vi "main.vi"() -> ()   [LabVIEW 2020]
uses:
  <vilib>/vision/Image Controls.llb/IMAQ Image.ctl
panel:
  in  "write buffer":string
  in  "TestBaud":u32=115200
  in  "TestPort":refnum<visa-resource-name>="COM6"
  out "TestReceivingFromSTM":string
  in  "Baud":u32=115200
  in  "Port":refnum<visa-resource-name>="COM6"
  out "ReceivingFromSTM":string
  in  "Recognise":bool
  in  "Process":bool
  in  "Stop acquisition":bool
  in  "Acquire":bool
  out "Image":T1(plugin-control)
  in  "Stop program":bool
  # "Serwo_Test"
  # "First Press \"Acquire\""
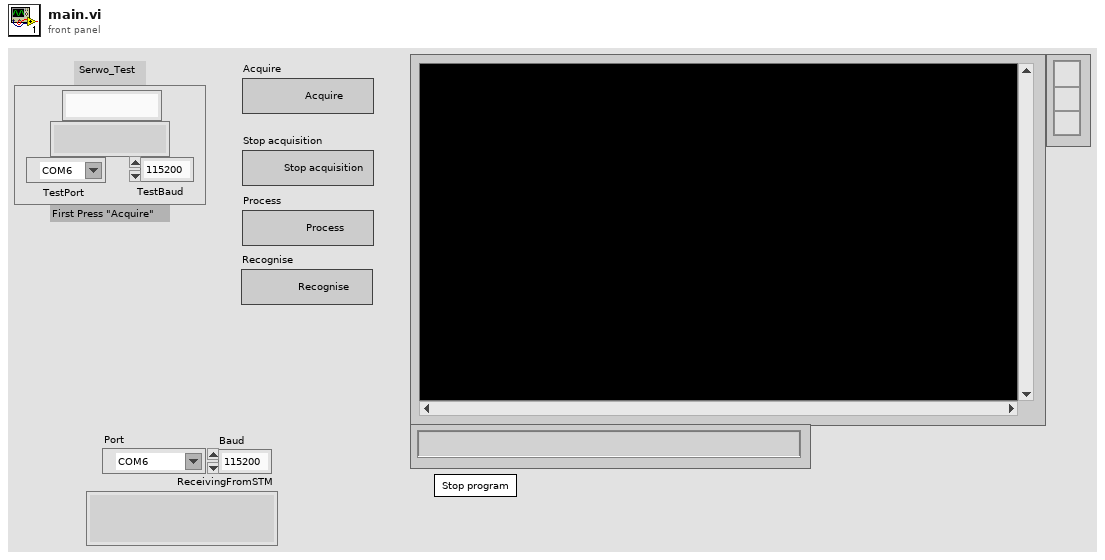
[diagram p1: front panel]
types:
  T1 = typedef "IMAQ Image.ctl" = refnum<image>
  T2 = enum32{"Invalid", "Standard", "Closed", "Hidden", "Minimized", "Maximized"}
  T3 = enum32{"invalid app kind", "Development System", "Run Time System", "Student Edition", "Embedded LabVIEW", "Evaluation", "Custom"}
  T4 = cluster{"Core":cluster{"Current VI Reference":refnum<vi>, "Close Panel on Exit?":bool}, "Aborted":bool, "New Image":T1, "Processing":bool, "Recognising":bool}
  T5 = cluster{"Current VI Reference":refnum<vi>, "Close Panel on Exit?":bool}
  T6 = typedef "Image Type" = u32
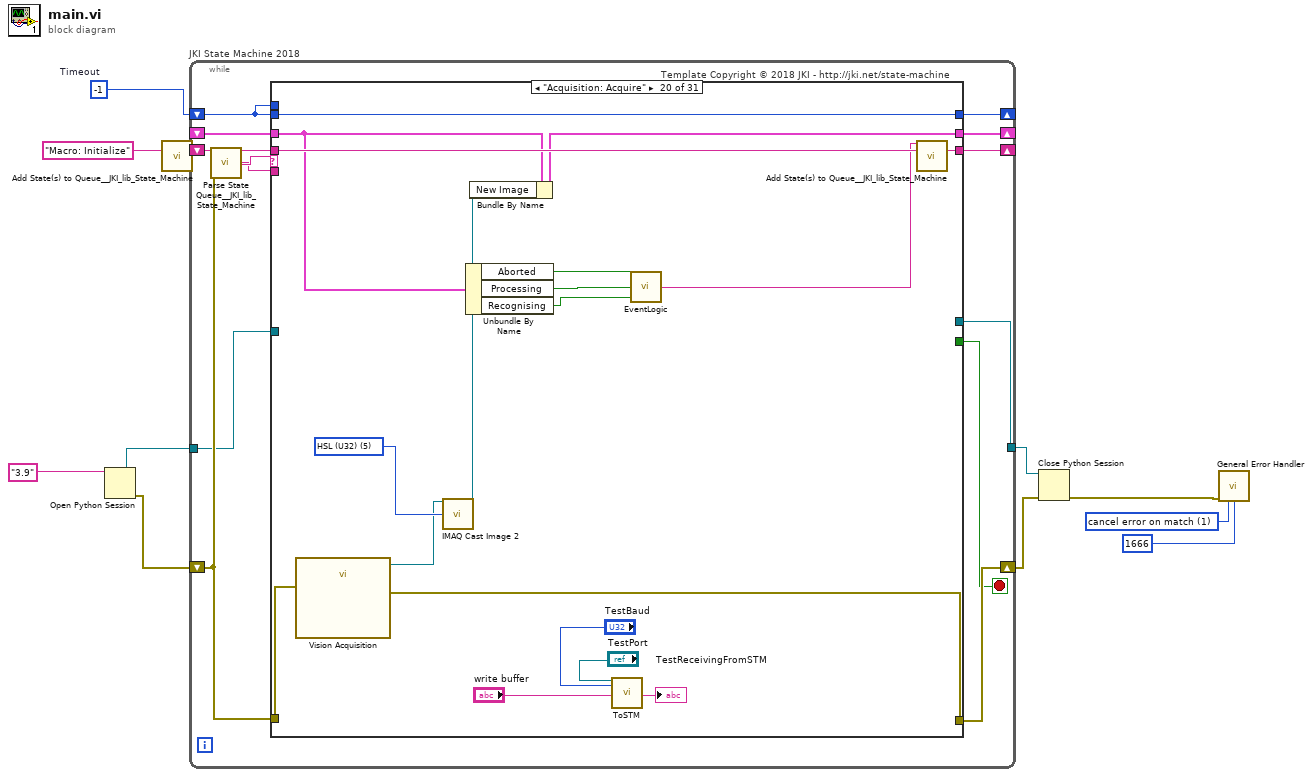
[diagram p0: block diagram]
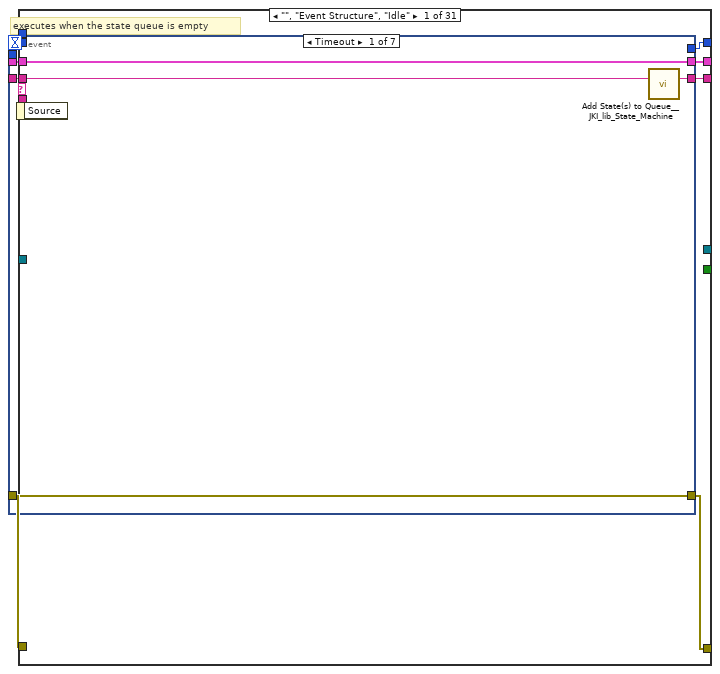
[diagram p2: hidden frame]
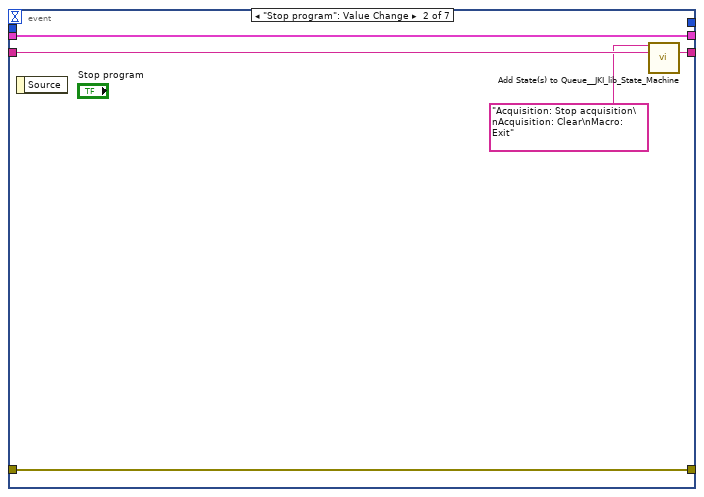
[diagram p3: hidden frame]
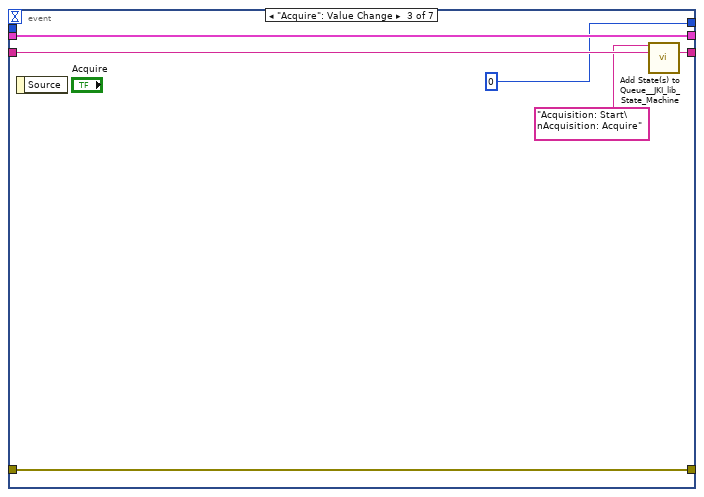
[diagram p4: hidden frame]
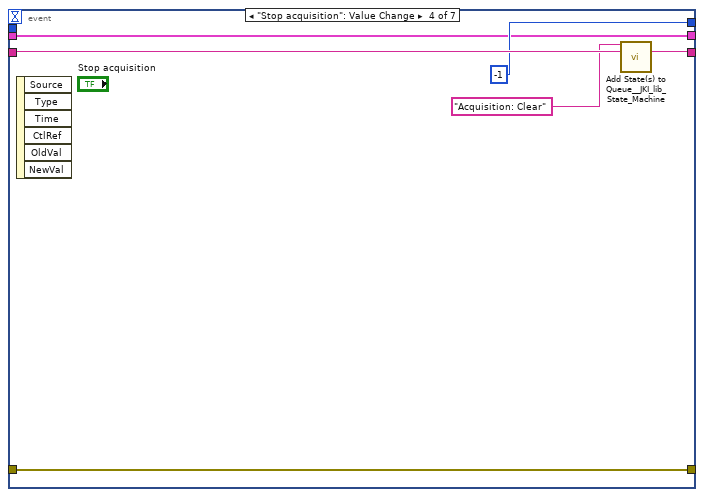
[diagram p5: hidden frame]
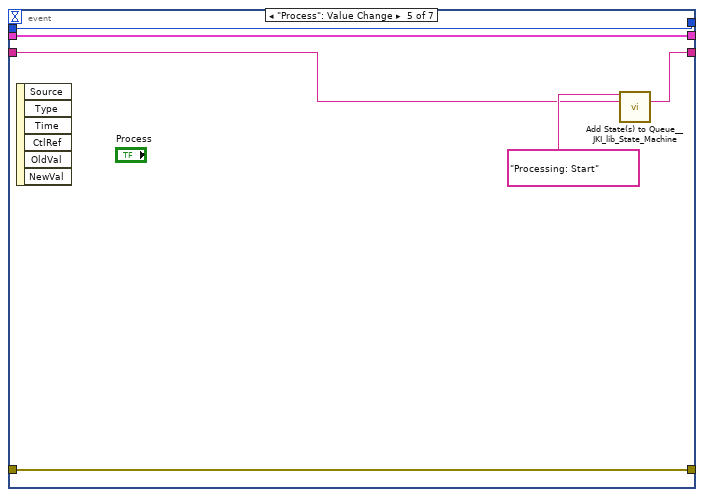
[diagram p6: hidden frame]
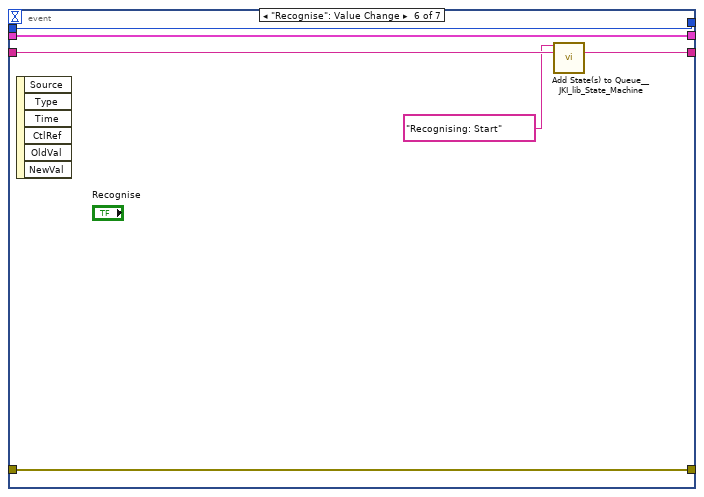
[diagram p7: hidden frame]
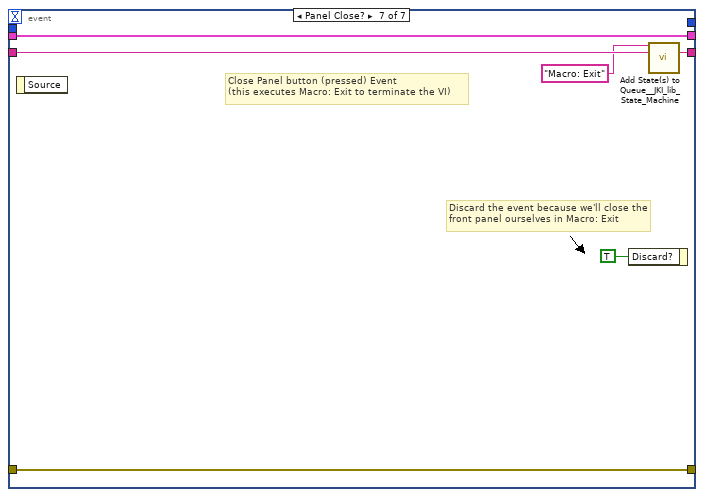
[diagram p8: hidden frame]
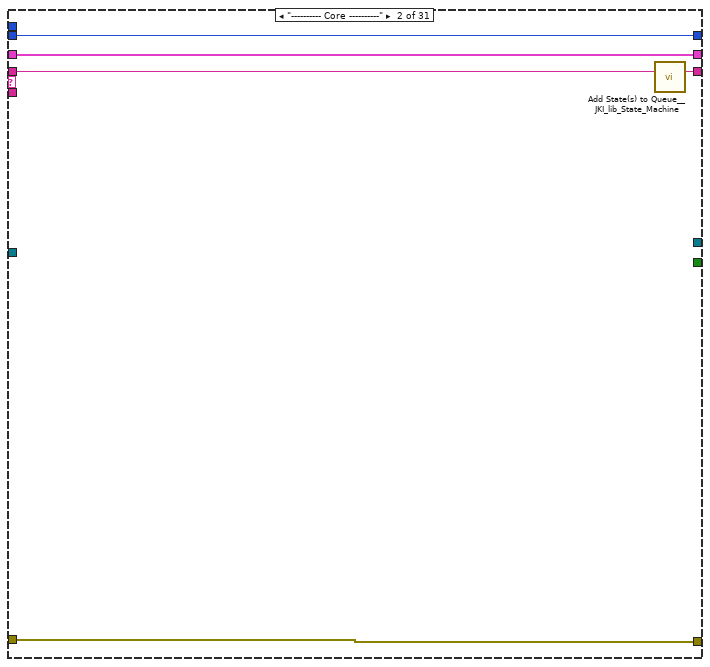
[diagram p9: hidden frame]
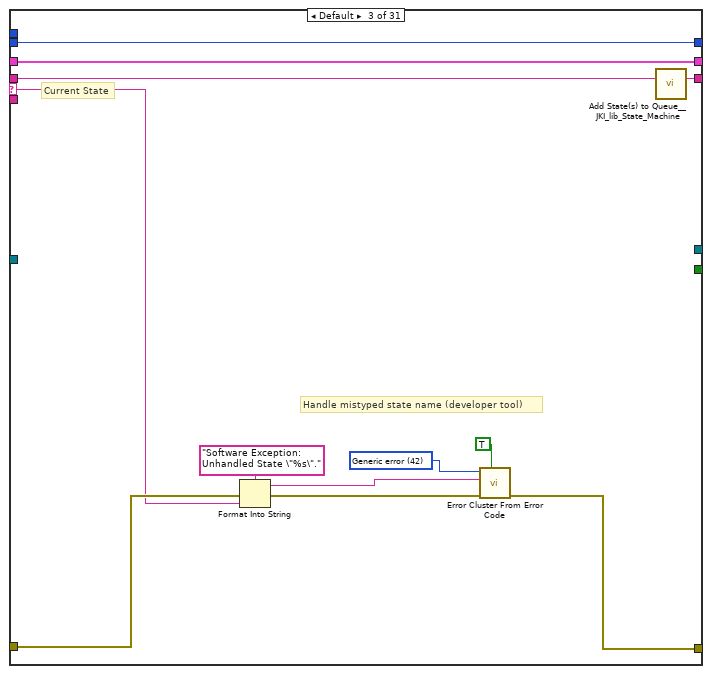
[diagram p10: hidden frame]
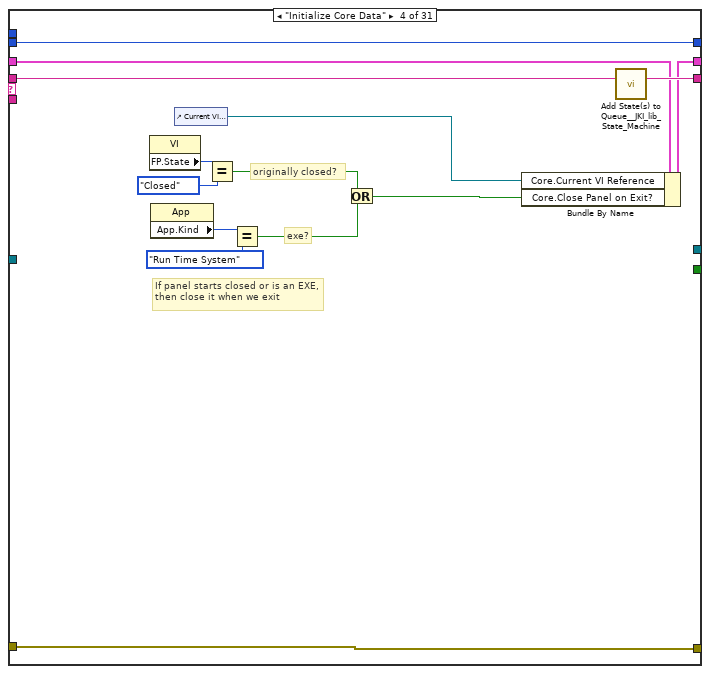
[diagram p11: hidden frame]
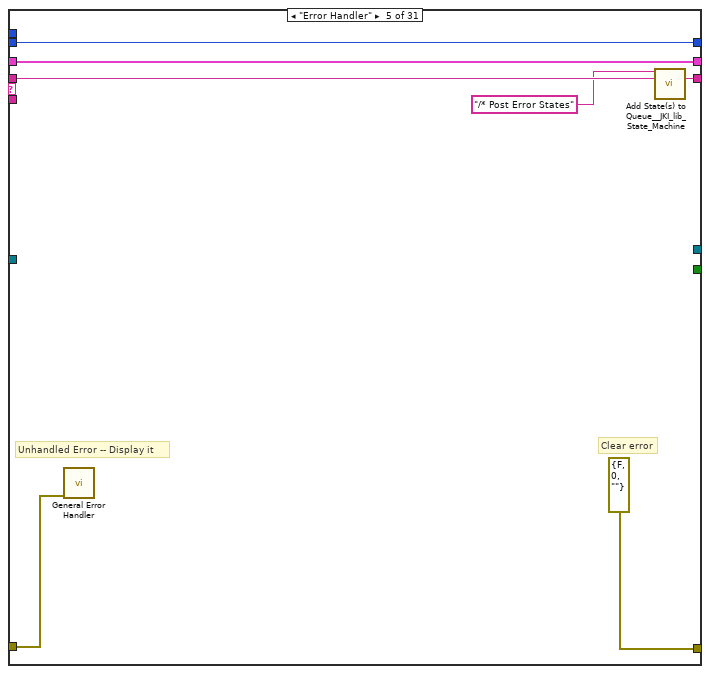
[diagram p12: hidden frame]
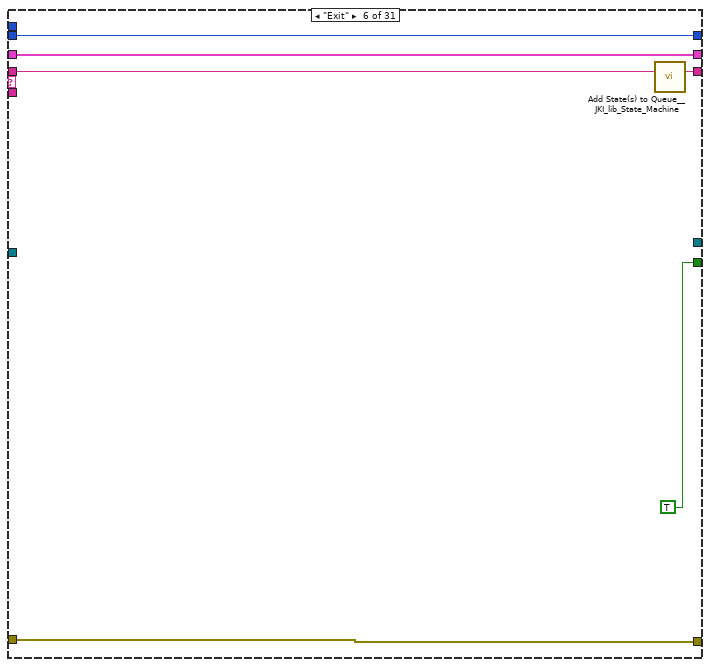
[diagram p13: hidden frame]
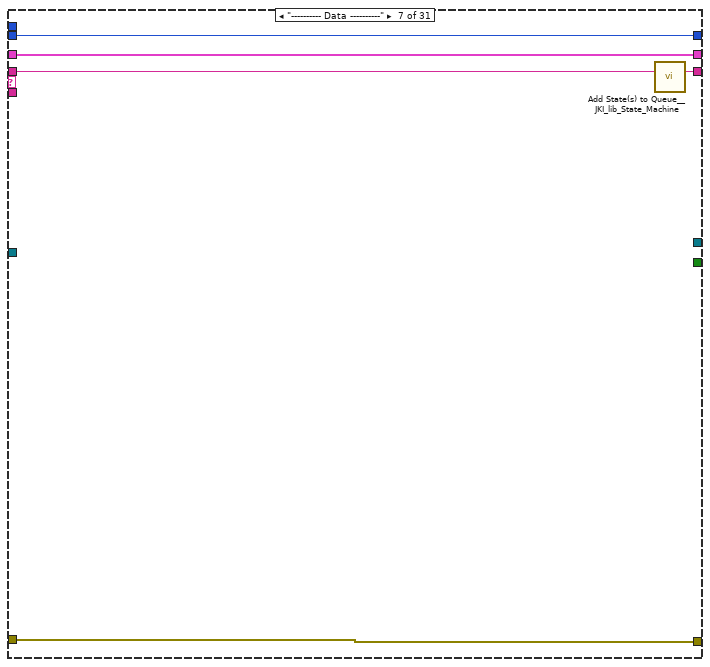
[diagram p14: hidden frame]
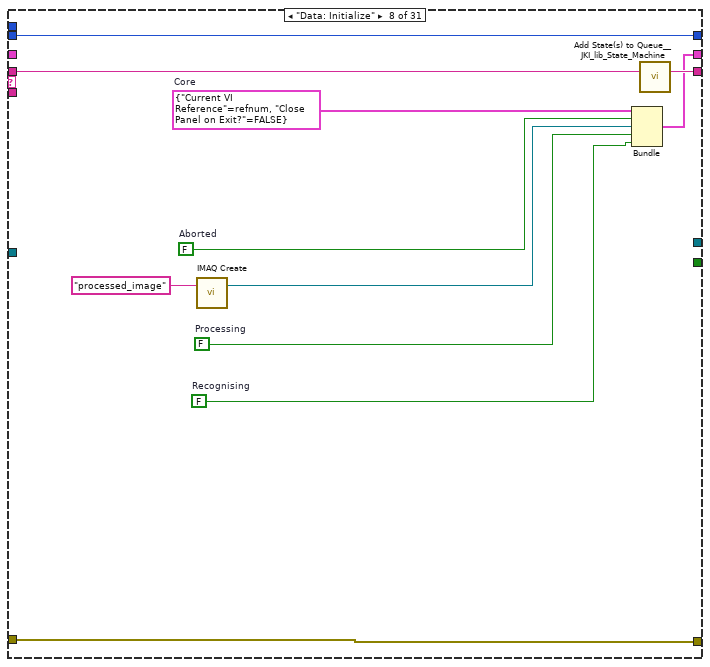
[diagram p15: hidden frame]
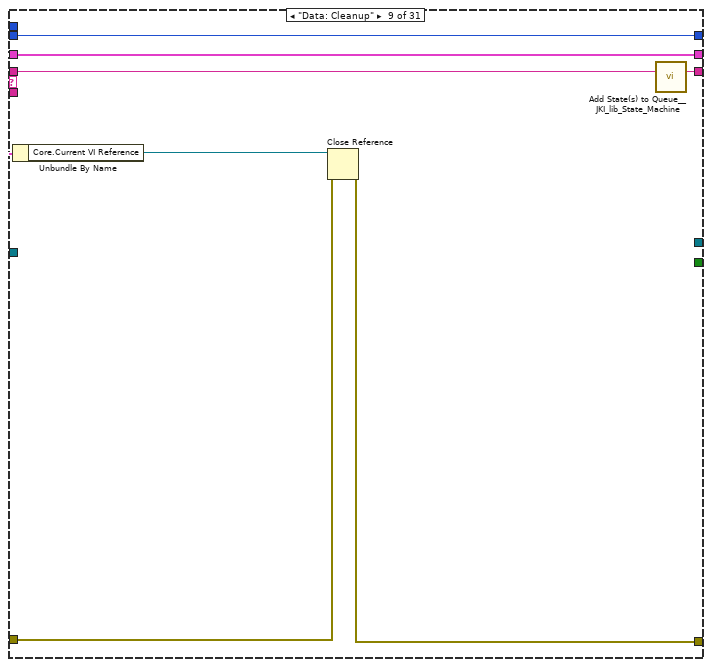
[diagram p16: hidden frame]
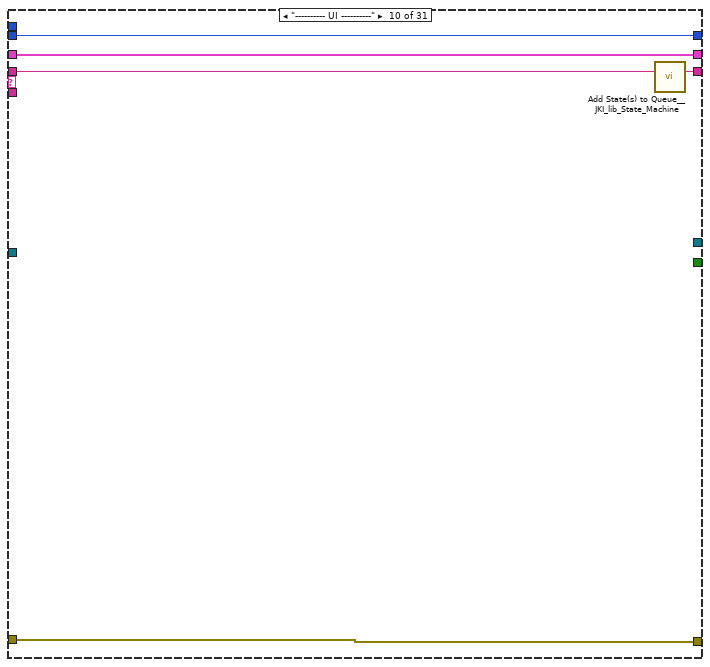
[diagram p17: hidden frame]
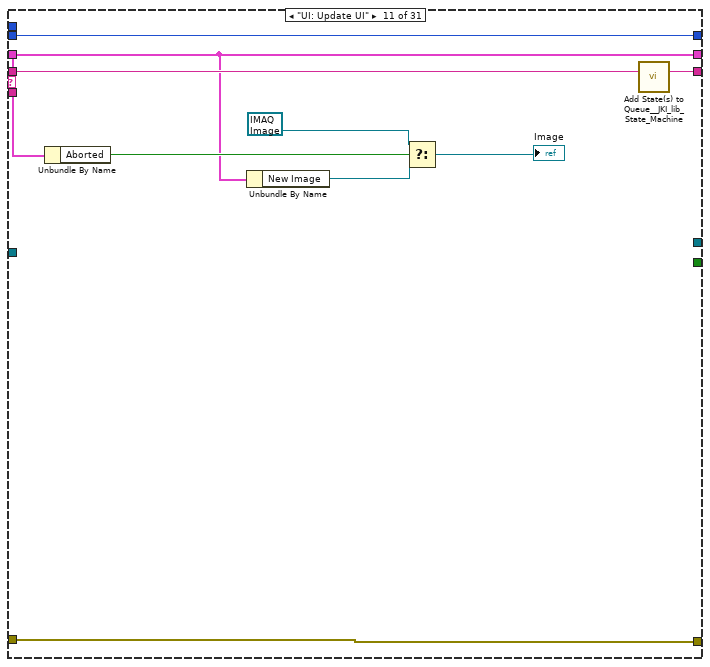
[diagram p18: hidden frame]
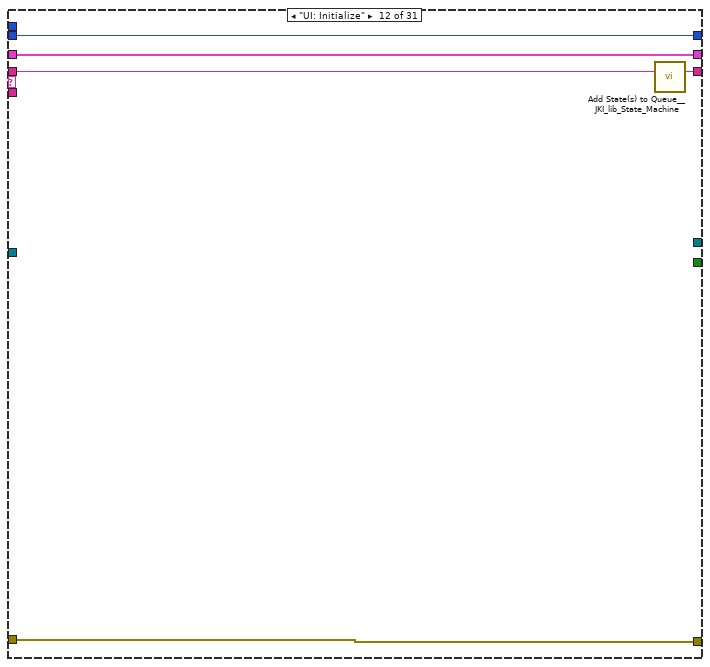
[diagram p19: hidden frame]
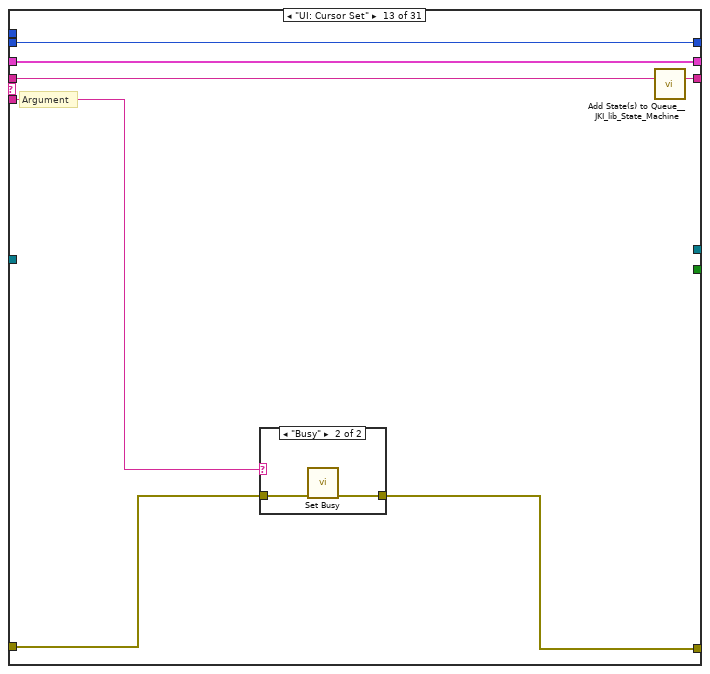
[diagram p20: hidden frame]
diagram:
  w3 = 1 items=["no exception", "cancel error on match", "set error on match"] ("[exception action] (none:0)")
  w9 = -1  # Timeout
  n1 = Open Python Session(python version="3.9" ("Python version")) -> (session out=w8:refnum<k35>, error out=w6:errorcluster)  [unwired: 2 in]
  n2 = call <vilib>:"Add State(s) to Queue__JKI_lib_State_Machine.vi"("State(s) in (\"\")"="Macro: Initialize") -> ("States Out"=w11:string)  [unwired: 14 in]
  n3 = while "JKI State Machine 2018" {
    shift-right: [w18] -> _
    shift-left: _ -> [w17]
    shift-right: [w21] -> w4
    shift-left: w6 -> [w16]
    shift-right: [w20] -> _
    shift-left: w11 -> [w22]
    shift-right: [w15] -> _
    shift-left: w9 -> [w14]
    tunnel: w8 -> [w13]
    tunnel: [w12] -> w5
    stop <- w19 stop-if-true
    # "Template Copyright © 2018 JKI - http://jki.net/state-machine"
    n4 = call <vilib>:"Parse State Queue__JKI_lib_State_Machine.vi"("State Queue"=w22, "Error In (no error)"=w16) -> ("Remaining States"=w24:string, "Current State"=w25:string, "Arguments"=w23:string)  [unwired: 11 in]
    n5 = case shown="\"Acquisition: Acquire\"" w25 {
      selector: w25 -> [_ _ w79 _ _ _ _ _ _ _ _ _ _ _ _ _ _ _ _ _ _ _ _ _ _ _ _ _ _ _ _]
      tunnel: w24 -> [w33 w77 w83 w103 w110 w116 w121 w132 w139 w144 w152 w158 w165 w177 w247 w253 w264 w269 w276 w294 w301 w310 w315 w320 w327 w347 w352 w357 w364 w386 w391]
      tunnel: w23 -> [_ _ _ _ _ _ _ _ _ _ _ _ w160 w171 _ _ _ _ _ _ _ _ _ _ _ _ _ _ _ _ _]
      tunnel: w17 -> [w31 w74 w81 w96 w107 w114 w118 _ w134 w141 w148 w156 w163 w173 w244 w250 w261 w266 w271 w292 w297 w306 w312 w317 w323 w343 w349 w354 w360 w371 w388]
      tunnel: [w30 w75 w85 w100 errorcluster {"status"=FALSE, "code"=0, "source"=""} ("error out") w113 w119 w129 w135 w142 w146 w155 w161 w174 w245 w251 w262 w267 w274 w286 w299 w308 w313 w318 w325 w336 w350 w355 w362 w370 w389] -> w21
      tunnel: w16 -> [w29 w75 w84 w100 w106 w113 w119 w129 w136 w142 w146 w155 w162 w175 w245 w251 w262 w267 w274 w282 w299 w308 w313 w318 w325 w335 w350 w355 w362 w373 w389]
      tunnel: [w32 w76 w82 w102 w109 w115 w120 w131 w138 w143 w153 w157 w164 w176 w246 w252 w263 w268 w275 w293 w300 w309 w314 w319 w326 w346 w351 w356 w363 w385 w390] -> w20
      tunnel: [_ _ _ _ _ TRUE _ _ _ _ _ _ _ _ _ _ _ _ _ _ _ _ _ _ _ _ _ _ _ _ _] -> w19
      tunnel: [w28 w74 w81 w101 w107 w114 w118 w130 w134 w141 w148 w156 w163 w173 w244 w250 w261 w266 w272 w291 w296 w306 w312 w317 w322 w342 w349 w354 w359 w371 w388] -> w18
      tunnel: w14 -> [w26 w73 _ w90 w104 w111 w117 w125 w133 w140 w145 w154 w159 w170 w243 w248 w254 w265 w270 w287 w298 w307 w311 w316 w324 w345 w348 w353 w361 w384 w387]
      tunnel: [w27 w73 w78 w90 w104 w111 w117 w125 w133 w140 w145 w154 w159 w170 w243 w248 w254 w265 w270 w287 w298 w307 w311 w316 w324 w345 w348 w353 w361 w384 w387] -> w15
      tunnel: w14 -> [_ _ w78 _ _ _ _ _ _ _ _ _ _ _ _ _ _ _ _ _ _ _ _ _ _ _ _ _ _ _ _]
      tunnel: w13 -> [_ _ _ _ _ _ _ _ _ _ _ _ _ _ _ _ _ _ _ _ _ _ _ _ _ w329 _ _ _ w372 _]
      tunnel: [_ _ _ _ _ _ _ _ _ _ _ _ _ _ _ _ _ _ _ _ _ _ _ _ _ w328 _ _ _ w368 _] -> w12
      frame "", "Event Structure", "Idle" {
        # "executes when the state queue is empty"
        n6 = event shown="[0] Timeout" {
          selector: _ -> [_ _ _ _ _ _ _]
          dyn-events: _ -> [_ _ _ _ _ _ _]
          timeout: w26 -> [_ _ _ _ _ _ _]
          tunnel: w33 -> [w37 w42 w48 w53 w55 w65 w72]
          tunnel: [w36 w41 w47 w54 w59 w63 w71] -> w32
          tunnel: w31 -> [w34 w39 w45 w50 w60 w66 w69]
          tunnel: [w35 w40 w46 w49 w56 w62 w70] -> w30
          tunnel: w29 -> [w35 w40 w46 w49 w56 w62 w70]
          tunnel: [w34 w39 w45 w50 w60 w66 w69] -> w28
          tunnel: [_ _ 0 ("Timeout") -1 ("Timeout") w57 w61 _] -> w27
          tunnel: w26 -> [_ _ _ _ w57 w61 _]
          event Timeout {
            n7 = event-data() -> ()  [unwired: 1 in, 1 out]
            n8 = call <vilib>:"Add State(s) to Queue__JKI_lib_State_Machine.vi"("State(s) in (\"\")"=w37) -> ("States Out"=w36:string)  [unwired: 14 in]
          }
          event "Stop program": Value Change {
            n9 = event-data() -> ()  [unwired: 1 in, 1 out]
            n10 = call <vilib>:"Add State(s) to Queue__JKI_lib_State_Machine.vi"("State(s) in Front (\"\")"="Acquisition: Stop acquisition\nAcquisition: Clear\nMacro: Exit", "State(s) in (\"\")"=w42) -> ("States Out"=w41:string)  [unwired: 13 in]
          }
          event "Acquire": Value Change {
            n11 = event-data() -> ()  [unwired: 1 in, 1 out]
            n12 = call <vilib>:"Add State(s) to Queue__JKI_lib_State_Machine.vi"("State(s) in Front (\"\")"="Acquisition: Start\nAcquisition: Acquire", "State(s) in (\"\")"=w48) -> ("States Out"=w47:string)  [unwired: 13 in]
          }
          event "Stop acquisition": Value Change {
            n13 = event-data() -> ()  [unwired: 1 in, 6 out]
            n14 = call <vilib>:"Add State(s) to Queue__JKI_lib_State_Machine.vi"("State(s) in Front (\"\")"="Acquisition: Clear" ("State(s) in Front (\"\")"), "State(s) in (\"\")"=w53) -> ("States Out"=w54:string)  [unwired: 13 in]
          }
          event "Process": Value Change {
            n15 = event-data() -> ()  [unwired: 1 in, 6 out]
            n16 = call <vilib>:"Add State(s) to Queue__JKI_lib_State_Machine.vi"("State(s) in Front (\"\")"="Processing: Start" ("State(s) in Front (\"\")"), "State(s) in (\"\")"=w55) -> ("States Out"=w59:string)  [unwired: 13 in]
          }
          event "Recognise": Value Change {
            n17 = event-data() -> ()  [unwired: 1 in, 6 out]
            n18 = call <vilib>:"Add State(s) to Queue__JKI_lib_State_Machine.vi"("State(s) in Front (\"\")"="Recognising: Start" ("State(s) in Front (\"\")"), "State(s) in (\"\")"=w65) -> ("States Out"=w63:string)  [unwired: 13 in]
          }
          event Panel Close? {
            # "Discard the event because we'll close the front panel ourselves in Macro: Exit"
            # "Close Panel button (pressed) Event\n(this executes Macro: Exit to terminate the VI)"
            n19 = event-data() -> ()  [unwired: 1 in, 1 out]
            n20 = event-data("Discard?"=TRUE) -> ()  [unwired: 1 in, 1 out]
            n21 = call <vilib>:"Add State(s) to Queue__JKI_lib_State_Machine.vi"("State(s) in Front (\"\")"="Macro: Exit", "State(s) in (\"\")"=w72) -> ("States Out"=w71:string)  [unwired: 13 in]
          }
        }
      }
      frame "---------- Core ----------" {
        n22 = call <vilib>:"Add State(s) to Queue__JKI_lib_State_Machine.vi"("State(s) in (\"\")"=w77) -> ("States Out"=w76:string)  [unwired: 14 in]
      }
      frame Default {
        w88 = 42 items=["No error", "Argument error", "Memory is full", "Out of zone", "End of file", "File already open", "Generic file I/O error", "File not found", "File permission error", "Disk is full", "Duplicate path", "Too many files open", "System feature not enabled", "Resource file not found", "Cannot add resource", "Resource not found", "Image not found", "Image memory error", "Pen does not exist", "Config type invalid", "Config token not found", "Config parse error", "Config memory error", "Bad external code format", "Bad external code offset", "External code not present", "Null window", "Destroy window error", "Null menu", "Print aborted", "Bad print record", "Print driver error", "Windows error during printing", "Memory error during printing", "Print dialog error", "Generic print error", "Invalid device refnum", "Device not found", "Device parameter error", "Device unit error", "Cannot open device", "Device call aborted", "Generic error", "Cancelled by user", "Object ID too low", "Object ID too high", "Object not in heap", "Unknown heap", "Unknown object (invalid DefProc)", "Unknown object (DefProc not in table)", "Message out of range", "Invalid (null) method", "Unknown message", "Manager call not supported", "Bad address", "Network operation in progress", "Network operation timed out", "Connection is busy", "Network attribute not supported", "Network error", "Address in use", "System out of memory", "Connection aborted", "Connection refused", "Not connected", "Already connected", "Connection closed", "Initialization error (interapplication manager)", "Bad occurrence", "Wait on unbound occurrence handler", "Occurrence queue overflow", "Datalog type conflict", "Unused", "Unrecognized type (interapplication manager)", "Memory corrupt", "Failed to make temporary DLL", "Old CIN version", "Drag socket not found", "Failed to load drop-object", "Failed to register OLE object", "Failed to release OLE object", "Format specifier type mismatch", "Unknown format specifier", "Too few format specifiers", "Too many format specifiers", "Scan failed", "Newer CIN version", "Error converting to variant", "Runtime menu error", "Password tampered", "Variant attribute not found", "Incompatible variant data type", "Event data is not available", "Event Store is not present", "Occurrence is not found", "Event Queue is not created", "Event info is not available", "Refnum passed is NULL", "Error retrieving Class GUID", "Error retrieving CoClass GUID", "Error retrieving TypeLib GUID.", "Bad built application magic bytes.", "Specific driver is different from the specific driver associated with the Logical Name.", "There is no session opened to the class driver.", "Max Error", "MAX - Error with config objects", "MAX - Error loading configuration", "MAX - Group not supported"]
        # "Current State"
        # "Handle mistyped state name (developer tool)"
        n23 = Format Into String(format string="Software Exception: Unhandled State \"%s\"." ("message"), error in=w84, w79) -> (resulting string=w87:string, error out=w86:errorcluster)  [unwired: 1 in]
        n24 = call <vilib>:"Error Cluster From Error Code.vi"("show call chain? (False)"=TRUE, "error in (no error)"=w86, "error message (\"\")"=w87, "error code (0)"=w88) -> ("error out"=w85:errorcluster)  [unwired: 5 in]
        n25 = call <vilib>:"Add State(s) to Queue__JKI_lib_State_Machine.vi"("State(s) in (\"\")"=w83) -> ("States Out"=w82:string)  [unwired: 14 in]
      }
      frame "Initialize Core Data" {
        # "originally closed?"
        # "exe?"
        # "If panel starts closed or is an EXE, then close it when we exit"
        n26 = property class="VI"() -> ("FP.State"=w93:T2)  [unwired: 2 in, 2 out]
        n27 = property class="App"() -> ("App.Kind"=w99:T3)  [unwired: 2 in, 2 out]
        n28 = control-ref of="Current VI Reference"() -> (w94:refnum<vi>)
        n29 = Equal?(x=w93, y=T2."Closed" ("Front Panel Window:State")) -> (x = y?=w91:bool)
        n30 = Equal?(x=w99, y=T3."Run Time System" ("Application:Kind")) -> (x = y?=w97:bool)
        n31 = Or(x=w91, y=w97) -> (x .or. y?=w95:bool)
        n32 = Bundle By Name(cluster=w96, "Core.Current VI Reference"=w94, "Core.Close Panel on Exit?"=w95) -> (w101:T4)
        n33 = call <vilib>:"Add State(s) to Queue__JKI_lib_State_Machine.vi"("State(s) in (\"\")"=w103) -> ("States Out"=w102:string)  [unwired: 14 in]
      }
      frame "Error Handler" {
        # "Unhandled Error -- Display it"
        # "Clear error"
        n34 = call <vilib>:"General Error Handler.vi"("error in (no error)"=w106) -> ()  [unwired: 10 in, 5 out]
        n35 = call <vilib>:"Add State(s) to Queue__JKI_lib_State_Machine.vi"("State(s) in Front (\"\")"="/* Post Error States", "State(s) in (\"\")"=w110) -> ("States Out"=w109:string)  [unwired: 13 in]
      }
      frame "Exit" {
        n36 = call <vilib>:"Add State(s) to Queue__JKI_lib_State_Machine.vi"("State(s) in (\"\")"=w116) -> ("States Out"=w115:string)  [unwired: 14 in]
      }
      frame "---------- Data ----------" {
        n37 = call <vilib>:"Add State(s) to Queue__JKI_lib_State_Machine.vi"("State(s) in (\"\")"=w121) -> ("States Out"=w120:string)  [unwired: 14 in]
      }
      frame "Data: Initialize" {
        w122 = FALSE  # Recognising
        w124 = FALSE  # Processing
        w123 = T5 {"Current VI Reference"=refnum, "Close Panel on Exit?"=FALSE}  # Core
        w128 = FALSE  # Aborted
        n38 = call "IMAQ Create"("Image Name"="processed_image") -> ("New Image"=w127:T1)  [unwired: 4 in, 1 out]
        n39 = Bundle("Core"=w123, "Aborted"=w128, "New Image"=w127, "Processing"=w124, "Recognising"=w122) -> (w130:T4)  [unwired: 1 in]
        n40 = call <vilib>:"Add State(s) to Queue__JKI_lib_State_Machine.vi"("State(s) in (\"\")"=w132) -> ("States Out"=w131:string)  [unwired: 14 in]
      }
      frame "Data: Cleanup" {
        n41 = Unbundle By Name(w134) -> ("Core.Current VI Reference"=w137:refnum<vi>)
        n42 = Close Reference(reference=w137, error in (no error)=w136) -> (error out=w135:errorcluster)
        n43 = call <vilib>:"Add State(s) to Queue__JKI_lib_State_Machine.vi"("State(s) in (\"\")"=w139) -> ("States Out"=w138:string)  [unwired: 14 in]
      }
      frame "---------- UI ----------" {
        n44 = call <vilib>:"Add State(s) to Queue__JKI_lib_State_Machine.vi"("State(s) in (\"\")"=w144) -> ("States Out"=w143:string)  [unwired: 14 in]
      }
      frame "UI: Update UI" {
        n45 = Unbundle By Name(w148) -> ("Aborted"=w151:bool)
        n46 = Unbundle By Name(w148) -> ("New Image"=w149:T1)
        n47 = Select(t=T1 refnum, s=w151, f=w149) -> (s? t:f=→"Image":T1)
        n48 = call <vilib>:"Add State(s) to Queue__JKI_lib_State_Machine.vi"("State(s) in (\"\")"=w152) -> ("States Out"=w153:string)  [unwired: 14 in]
      }
      frame "UI: Initialize" {
        n49 = call <vilib>:"Add State(s) to Queue__JKI_lib_State_Machine.vi"("State(s) in (\"\")"=w158) -> ("States Out"=w157:string)  [unwired: 14 in]
      }
      frame "UI: Cursor Set" {
        # "Argument"
        n50 = case shown="\"Busy\"" w160 {
          tunnel: w162 -> [w167 w169]
          tunnel: [w166 w168] -> w161
          frame "Idle", Default {
            n51 = call <vilib>:"Unset Busy.vi"("error in (no error)"=w167) -> ("error out"=w166:errorcluster)  [unwired: 10 in]
          }
          frame "Busy" {
            n52 = call <vilib>:"Set Busy.vi"("error in (no error)"=w169) -> ("error out"=w168:errorcluster)  [unwired: 9 in, 1 out]
          }
        }
        n53 = call <vilib>:"Add State(s) to Queue__JKI_lib_State_Machine.vi"("State(s) in (\"\")"=w165) -> ("States Out"=w164:string)  [unwired: 14 in]
      }
      frame "UI: Front Panel State" {
        # "Argument"
        n54 = Unbundle By Name(w173) -> ("Core.Current VI Reference"=w172:refnum<vi>)
        n55 = case shown="\"Hidden\", \"Hide\"" w171 {
          tunnel: w175 -> [w183 w198 w209 w222 w235]
          tunnel: [w185 w199 w211 w224 w237] -> w174
          tunnel: w172 -> [w184 w196 w210 w223 w236]
          frame "Open", "Standard", Default {
            w178 = T2."Standard" ("State")
            n56 = property class="VI"(reference=w184, error in=w183) -> (reference out=w181:refnum<vi>, error out=w182:errorcluster, "FP.State"=w180:T2)
            n57 = Not Equal?(x=w180, y=w178) -> (x != y?=w179:bool)
            n58 = case shown="True" w179 {
              tunnel: [w189 w191] -> w185
              tunnel: w182 -> [w188 w191]
              tunnel: w181 -> [w187 _]
              tunnel: w178 -> [w186 _]
              frame True {
                n59 = invoke class="VI" method="FP.Open"(reference=w187, error in=w188, "Activate"=TRUE, "State"=w186) -> (error out=w189:errorcluster)  [unwired: 1 in, 4 out]
              }
              frame False {
              }
            }
          }
          frame "Close", "Closed" {
            n60 = property class="VI"(reference=w196, error in=w198) -> (reference out=w195:refnum<vi>, error out=w197:errorcluster, "FP.State"=w193:T2)
            n61 = Not Equal?(x=w193, y=T2."Closed" ("Front Panel Window:State")) -> (x != y?=w192:bool)
            n62 = case shown="True" w192 {
              tunnel: [w200 w203] -> w199
              tunnel: w197 -> [w200 w202]
              tunnel: w195 -> [_ w201]
              frame False {
              }
              frame True {
                n63 = invoke class="VI" method="FP.Close"(reference=w201, error in=w202) -> (error out=w203:errorcluster)  [unwired: 1 in, 2 out]
              }
            }
          }
          frame "Hidden", "Hide" {
            w204 = T2."Hidden" ("State")
            n64 = property class="VI"(reference=w210, error in=w209) -> (reference out=w207:refnum<vi>, error out=w208:errorcluster, "FP.State"=w206:T2)
            n65 = Not Equal?(x=w206, y=w204) -> (x != y?=w205:bool)
            n66 = case shown="True" w205 {
              tunnel: [w215 w216] -> w211
              tunnel: w208 -> [w214 w216]
              tunnel: w207 -> [w213 _]
              tunnel: w204 -> [w212 _]
              frame True {
                n67 = invoke class="VI" method="FP.Open"(reference=w213, error in=w214, "State"=w212) -> (error out=w215:errorcluster)  [unwired: 2 in, 4 out]
              }
              frame False {
              }
            }
          }
          frame "Minimize", "Minimized" {
            w217 = T2."Minimized" ("State")
            n68 = property class="VI"(reference=w223, error in=w222) -> (reference out=w220:refnum<vi>, error out=w221:errorcluster, "FP.State"=w219:T2)
            n69 = Not Equal?(x=w219, y=w217) -> (x != y?=w218:bool)
            n70 = case shown="True" w218 {
              tunnel: [w228 w229] -> w224
              tunnel: w221 -> [w227 w229]
              tunnel: w220 -> [w226 _]
              tunnel: w217 -> [w225 _]
              frame True {
                n71 = invoke class="VI" method="FP.Open"(reference=w226, error in=w227, "State"=w225) -> (error out=w228:errorcluster)  [unwired: 2 in, 4 out]
              }
              frame False {
              }
            }
          }
          frame "Maximize", "Maximized" {
            w230 = T2."Maximized" ("State")
            n72 = property class="VI"(reference=w236, error in=w235) -> (reference out=w233:refnum<vi>, error out=w234:errorcluster, "FP.State"=w232:T2)
            n73 = Not Equal?(x=w232, y=w230) -> (x != y?=w231:bool)
            n74 = case shown="True" w231 {
              tunnel: [w241 w242] -> w237
              tunnel: w234 -> [w240 w242]
              tunnel: w233 -> [w239 _]
              tunnel: w230 -> [w238 _]
              frame True {
                n75 = invoke class="VI" method="FP.Open"(reference=w239, error in=w240, "State"=w238) -> (error out=w241:errorcluster)  [unwired: 2 in, 4 out]
              }
              frame False {
              }
            }
          }
        }
        n76 = call <vilib>:"Add State(s) to Queue__JKI_lib_State_Machine.vi"("State(s) in (\"\")"=w177) -> ("States Out"=w176:string)  [unwired: 14 in]
      }
      frame "---------- Macro ----------" {
        n77 = call <vilib>:"Add State(s) to Queue__JKI_lib_State_Machine.vi"("State(s) in (\"\")"=w247) -> ("States Out"=w246:string)  [unwired: 14 in]
      }
      frame "Macro: Initialize" {
        n78 = call <vilib>:"Add State(s) to Queue__JKI_lib_State_Machine.vi"("State(s) in Front (\"\")"="Data: Initialize\nInitialize Core Data\nUI: Initialize\nUI: Front Panel State >> Open", "State(s) in (\"\")"=w253) -> ("States Out"=w252:string)  [unwired: 13 in]
      }
      frame "Macro: Exit" {
        n79 = Unbundle By Name(w261) -> ("Core.Close Panel on Exit?"=w260:bool)
        n80 = Select(t="UI: Front Panel State >> Close", s=w260, f="") -> (s? t:f=w257:string)
        n81 = call <vilib>:"Add State(s) to Queue__JKI_lib_State_Machine.vi"("State(s) in (\"\")"=w257, "State(s) at Back (\"\")"="Data: Cleanup\nExit") -> ("States Out"=w255:string)  [unwired: 13 in]
        n82 = call <vilib>:"Add State(s) to Queue__JKI_lib_State_Machine.vi"("State(s) in Front (\"\")"=w255, "State(s) in (\"\")"=w264) -> ("States Out"=w263:string)  [unwired: 13 in]
      }
      frame "---------- Acquisition ----------" {
        n83 = call <vilib>:"Add State(s) to Queue__JKI_lib_State_Machine.vi"("State(s) in (\"\")"=w269) -> ("States Out"=w268:string)  [unwired: 14 in]
      }
      frame "Acquisition: Start" {
        n84 = Bundle By Name(cluster=w271, "Aborted"=FALSE) -> (w272:T4)
        n85 = call <vilib>:"Add State(s) to Queue__JKI_lib_State_Machine.vi"("State(s) in (\"\")"=w276) -> ("States Out"=w275:string)  [unwired: 14 in]
      }
      frame "Acquisition: Acquire" {
        w289 = T6 5 items=["Grayscale (U8)", "Grayscale (I16)", "Grayscale (SGL)", "Complex (CSG)", "RGB (U32)", "HSL (U32)", "RGB (U64)", "Grayscale (U16)"] ("Image Type")
        n86 = call "Vision Acquisition"("error in"=w282) -> ("Image Out"=w288:T1, "error out"=w286:errorcluster)  [unwired: 24 in, 1 out]
        n87 = call "IMAQ Cast Image 2"("Image Src"=w288, "Image Type"=w289) -> ("Image Dst Out"=w290:T1)  [unwired: 12 in, 1 out]
        n88 = Unbundle By Name(w292) -> ("Aborted"=w281:bool, "Processing"=w280:bool, "Recognising"=w279:bool)
        n89 = Bundle By Name(cluster=w292, "New Image"=w290) -> (w291:T4)
        n90 = call "ToSTM.vi"("Port"="TestPort", "Baud"="TestBaud", "write buffer"="write buffer") -> ("read buffer"=→"TestReceivingFromSTM":string)  [unwired: 16 in]
        n91 = call "EventLogic.vi"("Recognising"=w279, "Processing"=w280, "Aborted"=w281) -> ("WhatToDo"=w278:string)
        n92 = call <vilib>:"Add State(s) to Queue__JKI_lib_State_Machine.vi"("State(s) in Front (\"\")"=w278, "State(s) in (\"\")"=w294) -> ("States Out"=w293:string)  [unwired: 13 in]
      }
      frame "Acquisition: Stop acquisition" {
        n93 = Bundle By Name(cluster=w297, "Aborted"=TRUE) -> (w296:T4)
        n94 = call <vilib>:"Add State(s) to Queue__JKI_lib_State_Machine.vi"("State(s) in (\"\")"=w301) -> ("States Out"=w300:string)  [unwired: 14 in]
      }
      frame "Acquisition: Clear" {
        n95 = Unbundle By Name(w306) -> ("Aborted"=w305:bool)
        n96 = Select(t="UI: Update UI", s=w305, f="Acquisition: Stop acquisition") -> (s? t:f=w303:string)
        n97 = call <vilib>:"Add State(s) to Queue__JKI_lib_State_Machine.vi"("State(s) in Front (\"\")"=w303, "State(s) in (\"\")"=w310) -> ("States Out"=w309:string)  [unwired: 13 in]
      }
      frame "Acquisition: OK" {
        n98 = call <vilib>:"Add State(s) to Queue__JKI_lib_State_Machine.vi"("State(s) in (\"\")"=w315) -> ("States Out"=w314:string)  [unwired: 14 in]
      }
      frame "---------- Processing ----------" {
        n99 = call <vilib>:"Add State(s) to Queue__JKI_lib_State_Machine.vi"("State(s) in (\"\")"=w320) -> ("States Out"=w319:string)  [unwired: 14 in]
      }
      frame "Processing: Start" {
        n100 = Bundle By Name(cluster=w323, "Processing"=TRUE ("IsFaceDetectionON")) -> (w322:T4)
        n101 = call <vilib>:"Add State(s) to Queue__JKI_lib_State_Machine.vi"("State(s) in (\"\")"=w327) -> ("States Out"=w326:string)  [unwired: 14 in]
      }
      frame "Processing: Process" {
        n102 = Unbundle By Name(w343) -> ("New Image"=w340:T1)
        n103 = call <vilib>:"Application Directory.vi"() -> ("Application Directory"=w332:path)
        n104 = call "IMAQ ColorImageToArray"("Image"=w340, "error in (no error)"=w335) -> ("Image Pixels (U32)"=w339:u32[][], "error out"=w334:errorcluster)  [unwired: 2 in, 1 out]
        n105 = Build Path(base path=w332, name or relative path="python\\process_image.py") -> (appended path=w331:path)
        n106 = node(w329, w331, "get_image" ("function name"), w334, w339, w339) -> (w328:refnum<k35>, w337:errorcluster, w338:u32[][])  [unwired: 1 in, 2 out]
        n107 = call "IMAQ ArrayToColorImage"("Image Pixels (U32)"=w338, "Image"=w340, "error in (no error)"=w337) -> ("Image Out"=w341:T1, "error out"=w336:errorcluster)  [unwired: 2 in]
        n108 = Bundle By Name(cluster=w343, "New Image"=w341) -> (w342:T4)
        n109 = call <vilib>:"Add State(s) to Queue__JKI_lib_State_Machine.vi"("State(s) in Front (\"\")"="UI: Update UI" ("State(s) in Front (\"\")"), "State(s) in (\"\")"=w347) -> ("States Out"=w346:string)  [unwired: 13 in]
      }
      frame "Processing: Ok" {
        n110 = call <vilib>:"Add State(s) to Queue__JKI_lib_State_Machine.vi"("State(s) in (\"\")"=w352) -> ("States Out"=w351:string)  [unwired: 14 in]
      }
      frame "---------- Recognising----------" {
        n111 = call <vilib>:"Add State(s) to Queue__JKI_lib_State_Machine.vi"("State(s) in (\"\")"=w357) -> ("States Out"=w356:string)  [unwired: 14 in]
      }
      frame "Recognising: Start" {
        n112 = Bundle By Name(cluster=w360, "Recognising"=TRUE ("IsFaceDetectionON")) -> (w359:T4)
        n113 = call <vilib>:"Add State(s) to Queue__JKI_lib_State_Machine.vi"("State(s) in (\"\")"=w364) -> ("States Out"=w363:string)  [unwired: 14 in]
      }
      frame "Recognising: Recognise" {
        n114 = Unbundle By Name(w371) -> ("New Image"=w379:T1)
        n115 = call <vilib>:"Application Directory.vi"() -> ("Application Directory"=w376:path)
        n116 = call "IMAQ ColorImageToArray"("Image"=w379, "error in (no error)"=w373) -> ("Image Pixels (U32)"=w369:u32[][], "error out"=w378:errorcluster)  [unwired: 2 in, 1 out]
        n117 = Build Path(base path=w376, name or relative path="python\\recognise_color.py") -> (appended path=w375:path)
        n118 = node(w372, w375, "get_image" ("function name"), w378, 0, w369) -> (w368:refnum<k35>, w370:errorcluster, w365:i32)  [unwired: 1 in, 2 out]
        n119 = Number To Decimal String(number=w365) -> (decimal integer string=w366:string)  [unwired: 1 in]
        n120 = call "ToSTM.vi"("Port"="Port", "Baud"="Baud", "write buffer"=w366) -> ("read buffer"=→"ReceivingFromSTM":string)  [unwired: 16 in]
        n121 = call <vilib>:"Add State(s) to Queue__JKI_lib_State_Machine.vi"("State(s) in Front (\"\")"="UI: Update UI" ("State(s) in Front (\"\")"), "State(s) in (\"\")"=w386) -> ("States Out"=w385:string)  [unwired: 13 in]
      }
      frame "Recognising: Ok" {
        n122 = call <vilib>:"Add State(s) to Queue__JKI_lib_State_Machine.vi"("State(s) in (\"\")"=w391) -> ("States Out"=w390:string)  [unwired: 14 in]
      }
    }
  }
  n123 = Close Python Session(session in=w5, error in=w4) -> (11:w1:errorcluster)
  n124 = call <vilib>:"General Error Handler.vi"("error in (no error)"=w1, "[exception action] (none:0)"=w3, "[exception code]"=1666) -> ()  [unwired: 8 in, 5 out]
